vi "FTW-CodeGen-FindGObjects-Callback.vi"(4 "context in":variant, 5 "objref":refnum<vi>) -> (1 "context out":variant, 2 "traverse flags":i32 format="0x%08x")   [LabVIEW 2014]
panel:
  # "Inputs"
  # "Outputs"
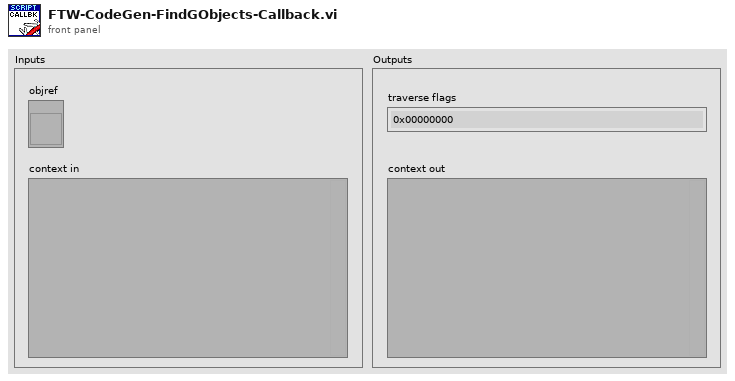
[diagram p1: front panel]
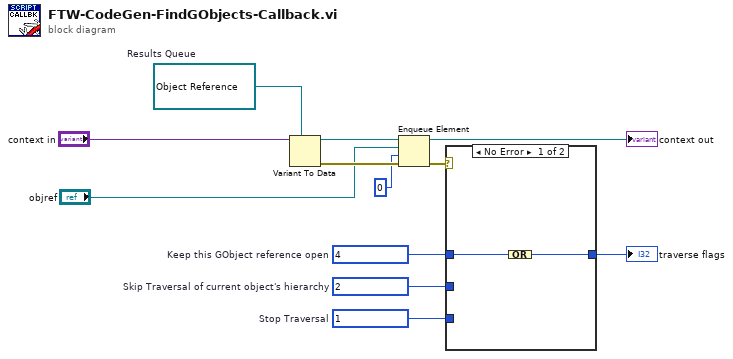
[diagram p0: block diagram]
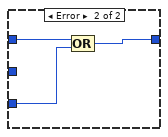
[diagram p2: hidden frame]
diagram:
  w10 = refnum<queue> refnum  # Results Queue
  w12 = 4  # Keep this GObject reference open
  w2 = 2  # Skip Traversal of current object's hierarchy
  w1 = 1  # Stop Traversal
  n1 = Variant To Data(type=w10, Variant="context in") -> (data=w8:refnum<queue>, error out=w7:errorcluster)  [unwired: 1 in]
  n2 = Enqueue Element(queue=w8, element="objref", timeout in ms (-1)=0, error in (no error)=w7) -> (queue out=→"context out":refnum<queue>, error out=w3:errorcluster)  [unwired: 1 out]
  n3 = case shown="No Error" w3 {
    tunnel: w12 -> [w14 w17]
    tunnel: [w13 w16] -> w11
    tunnel: w2 -> [_ _]
    tunnel: w1 -> [_ w15]
    frame No Error {
      n4 = Compound Arithmetic op=OR(w14) -> (w13:i32)
    }
    frame Error {
      n5 = Compound Arithmetic op=OR(w17, w15) -> (w16:i32)
    }
  }
  "traverse flags" <- w11
